vi "2ball.vi"() -> (3 "Outputs":T6)   [LabVIEW 2013]
uses:
  outputs.ctl
  drive/drive_outputs.ctl
  flinger/flinger_outputs.ctl
  <vilib>/Rock Robotics/WPI/Solenoid/WPI_SolenoidValue.ctl
  roller/roller_outputs.ctl
  catch/catch_outputs.ctl
  inputs.ctl
  drive/drive_inputs.ctl
  flinger/flinger_inputs.ctl
  roller/roller_inputs.ctl
  catch/catch_inputs.ctl
panel:
  in  "Inputs 2":T1
  in  "Inputs":T1
  in  "Outputs 2":T6
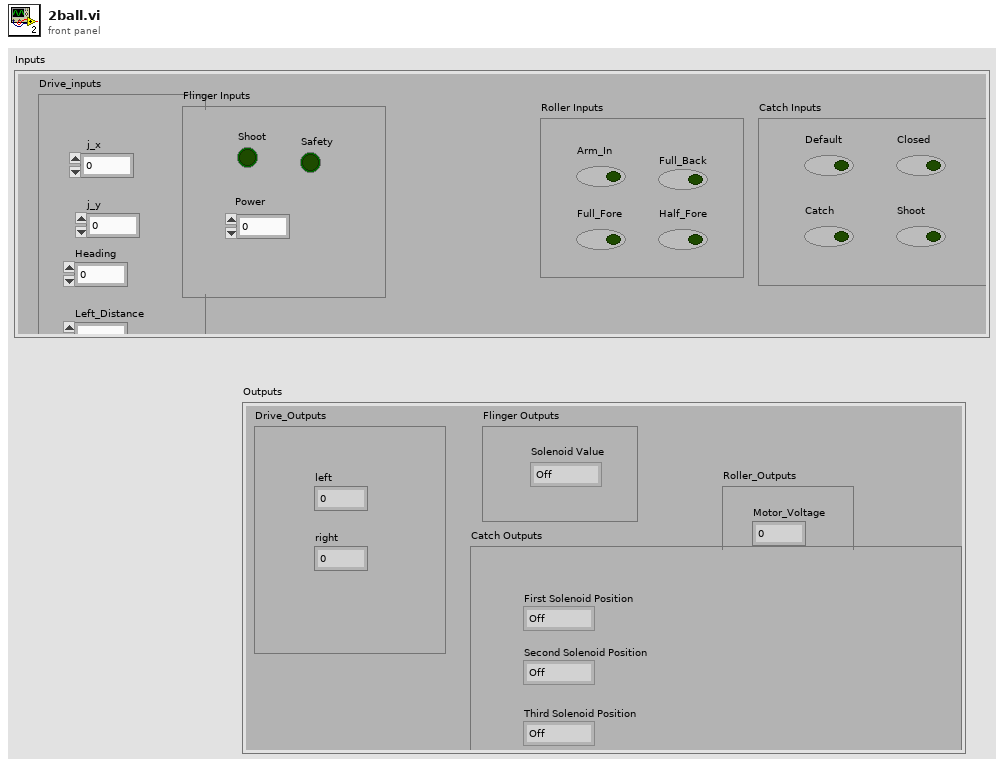
[diagram p1: front panel]
types:
  T1 = typedef "inputs.ctl" = cluster{"Drive_inputs":T2, "Flinger Inputs":T3, "Roller Inputs":T4, "Catch Inputs":T5}
  T2 = typedef "drive_inputs.ctl" = cluster{"j_x":dbl, "j_y":dbl, "Heading":dbl, "Left_Distance":dbl, " Right_Distance":dbl}
  T3 = typedef "flinger_inputs.ctl" = cluster{"Shoot":bool, "Power":dbl, "Safety":bool}
  T4 = typedef "roller_inputs.ctl" = cluster{"Arm_In":bool, "Full_Fore":bool, "Full_Back":bool, "Half_Fore":bool}
  T5 = typedef "catch_inputs.ctl" = cluster{"Default":bool, "Closed":bool, "Catch":bool, "Shoot":bool}
  T6 = typedef "outputs.ctl" = cluster{"Drive_Outputs":T7, "Flinger Outputs":T8, "Roller_Outputs":T10, "Catch Outputs":T11}
  T7 = typedef "drive_outputs.ctl" = cluster{"left":dbl, "right":dbl}
  T8 = typedef "flinger_outputs.ctl" = cluster{"Solenoid Value":T9}
  T9 = typedef "WPI_SolenoidValue.ctl" = enum16{"Off", "On", "Forward", "Reverse"}
  T10 = typedef "roller_outputs.ctl" = cluster{"Sol_Position":T9, "Motor_Voltage":dbl}
  T11 = typedef "catch_outputs.ctl" = cluster{"First Solenoid Position":T9, "Second Solenoid Position":T9, "Third Solenoid Position":T9}
  T12 = typedef "WPI_EncoderDevRef.ctl" = cluster{"DevStatus":errorcluster, "EncoderIndex":T13, "CounterIndex":T14, "DistancePerCount":dbl, "Decoding Type":T15}
  T13 = typedef "FPGA_EncoderIdx.ctl" = enum8{"Enc 0", "Enc 1", "Enc 2", "Enc 3", "Invalid"}
  T14 = typedef "FPGA_CounterCtrSystemIndex.ctl" = enum8{"Ctr 0", "Ctr 1", "Ctr 2", "Ctr 3", "Ctr 4", "Ctr 5", "Ctr 6", "Ctr 7", "Invalid"}
  T15 = typedef "WPI_EncoderType.ctl" = enum16{"1x", "2x", "4x"}
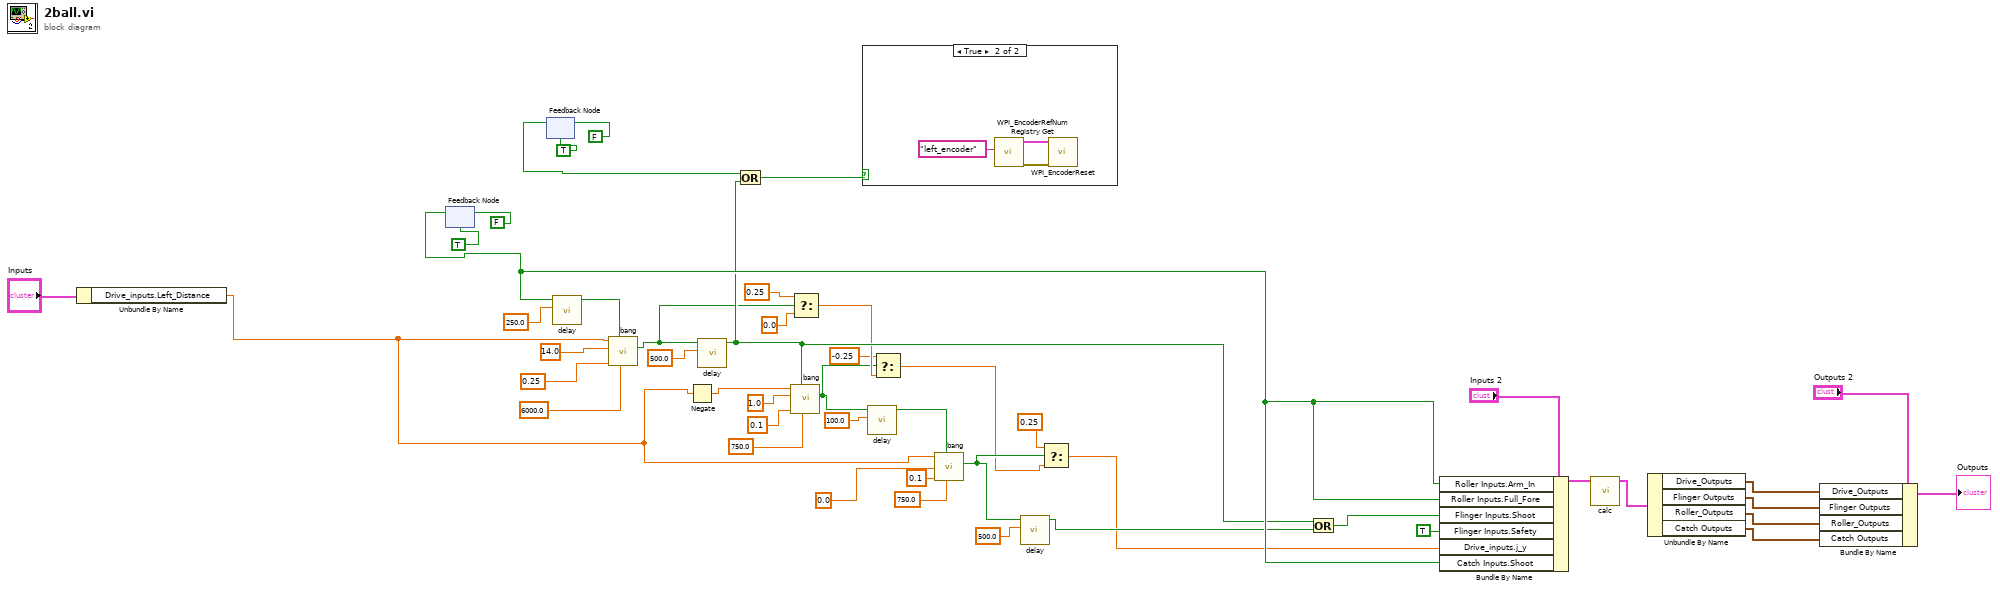
[diagram p0: block diagram]
diagram:
  n1 = Unbundle By Name("Inputs") -> ("Drive_inputs.Left_Distance"=w16:dbl)
  n2 = feedback #1(TRUE) -> (w15:bool)
  n3 = feedback-in #1(FALSE) -> ()
  n4 = feedback-in #2(FALSE) -> ()
  n5 = feedback #2(TRUE) -> (w21:bool)
  n6 = call "delay.vi"("Wait"=250.0, "In"=w15) -> ("Out"=w35:bool)  [unwired: 9 in]
  n7 = call "bang.vi"("Sanity"=6000.0, "Start"=w35, "Tolerance"=0.25, "Set"=14.0, "Pos"=w16) -> ("B_Out"=w10:bool)  [unwired: 6 in]
  n8 = Negate(x=w16) -> (-x=w17:dbl)
  n9 = call "delay.vi"("Wait"=500.0, "In"=w10) -> ("Out"=w11:bool)  [unwired: 9 in]
  n10 = Or(x=w21, y=w11) -> (x .or. y?=w20:bool)
  n11 = call "bang.vi"("Sanity"=750.0, "Start"=w11, "Tolerance"=0.1, "Set"=1.0, "Pos"=w17) -> ("B_Out"=w6:bool)  [unwired: 6 in]
  n12 = Select(t=0.25, s=w10, f=0.0) -> (s? t:f=w7:dbl)
  n13 = case shown="True" w20 {
    frame False {
    }
    frame True {
      n14 = call <vilib>:"WPI_EncoderRefNum Registry Get.vi"("refnum name"="left_encoder") -> ("error out"=w51:errorcluster, "EncoderDevRef"=w50:T12)  [unwired: 9 in]
      n15 = call <vilib>:"WPI_EncoderReset.vi"("error in (no error)"=w51, "EncoderDevRef"=w50) -> ()  [unwired: 8 in, 2 out]
    }
  }
  n16 = call "delay.vi"("Wait"=100.0, "In"=w6) -> ("Out"=w26:bool)  [unwired: 9 in]
  n17 = Select(t=-0.25, s=w6, f=w7) -> (s? t:f=w3:dbl)
  n18 = call "bang.vi"("Sanity"=750.0, "Start"=w26, "Tolerance"=0.1, "Set"=0.0, "Pos"=w16) -> ("B_Out"=w4:bool)  [unwired: 6 in]
  n19 = call "delay.vi"("Wait"=500.0, "In"=w4) -> ("Out"=w12:bool)  [unwired: 9 in]
  n20 = Select(t=0.25, s=w4, f=w3) -> (s? t:f=w1:dbl)
  n21 = Or(x=w11, y=w12) -> (x .or. y?=w13:bool)
  n22 = Bundle By Name(cluster="Inputs 2", "Roller Inputs.Arm_In"=w15, "Roller Inputs.Full_Fore"=w15, "Flinger Inputs.Shoot"=w13, "Flinger Inputs.Safety"=TRUE, "Drive_inputs.j_y"=w1, "Catch Inputs.Shoot"=w15) -> (w46:T1)
  n23 = call "calc.vi"("Inputs"=w46) -> ("Outputs"=w43:T6)  [unwired: 10 in]
  n24 = Unbundle By Name(w43) -> ("Drive_Outputs"=w42:T7, "Flinger Outputs"=w41:T8, "Roller_Outputs"=w40:T10, "Catch Outputs"=w39:T11)
  n25 = Bundle By Name(cluster="Outputs 2", "Drive_Outputs"=w42, "Flinger Outputs"=w41, "Roller_Outputs"=w40, "Catch Outputs"=w39) -> (→"Outputs":T6)
